vi "DropDetectionForLinkam.vi"(6 "Max(µm)":dbl min=0.0 format="%#_g µm", 7 "Min(µm)":dbl min=0.0 format="%#_g µm", 8 "error in":errorcluster, 9 "Mag":T1, 10 "Minimum match score":dbl=950.0, 11 "Image in":T4(plugin-control)) -> (0 "error out":errorcluster, 1 "Mag out":T1, 2 "Matches (pixel)":T3(array[cluster]), 3 "Image Out":T4(plugin-control), 4 "Circles (Calibrated)":T5(array[cluster]) {"Position"."Y" format="%.2f"; "Position"."X" format="%.2f"})   [LabVIEW 2013]
uses:
  Mag.ctl
  <vilib>/vision/NI_Vision_Development_Module.lvlib
  <vilib>/Analysis/NI_AALPro.lvlib
  <vilib>/Analysis/NI_AAL_SigProc.lvlib
panel:
  in  "Magnification (Microns/Pixel)":dbl(ring)=2.731524 items=["5x_M_BD"=2.731524, "10x_M"=1.3634, "10xM_BD"=1.3543, "10x_ph1"=1.3439, "20x_S"=0.68129, "20x_LM"=0.714285, "50x_S"=0.277777, "100x_im"=0.119047]
  out "fractional index or x":dbl
  out "XY Graph":cluster{i32[], "dX/dt":dbl[]}[](graph)
  in  "Annulus":T2 {"End Angle" min=-90.0 max=90.0 step=1.0 format="%.2f"; "Start Angle" min=-90.0 max=90.0 step=1.0 format="%.2f"; "Center X" scale=0.0..1024.0}
  in  "Circle Descriptor":cluster{"Min Radius":dbl, "Max Radius":dbl}={"Min Radius"=3.0, "Max Radius"=500.0}
  out "Number of matches":i32
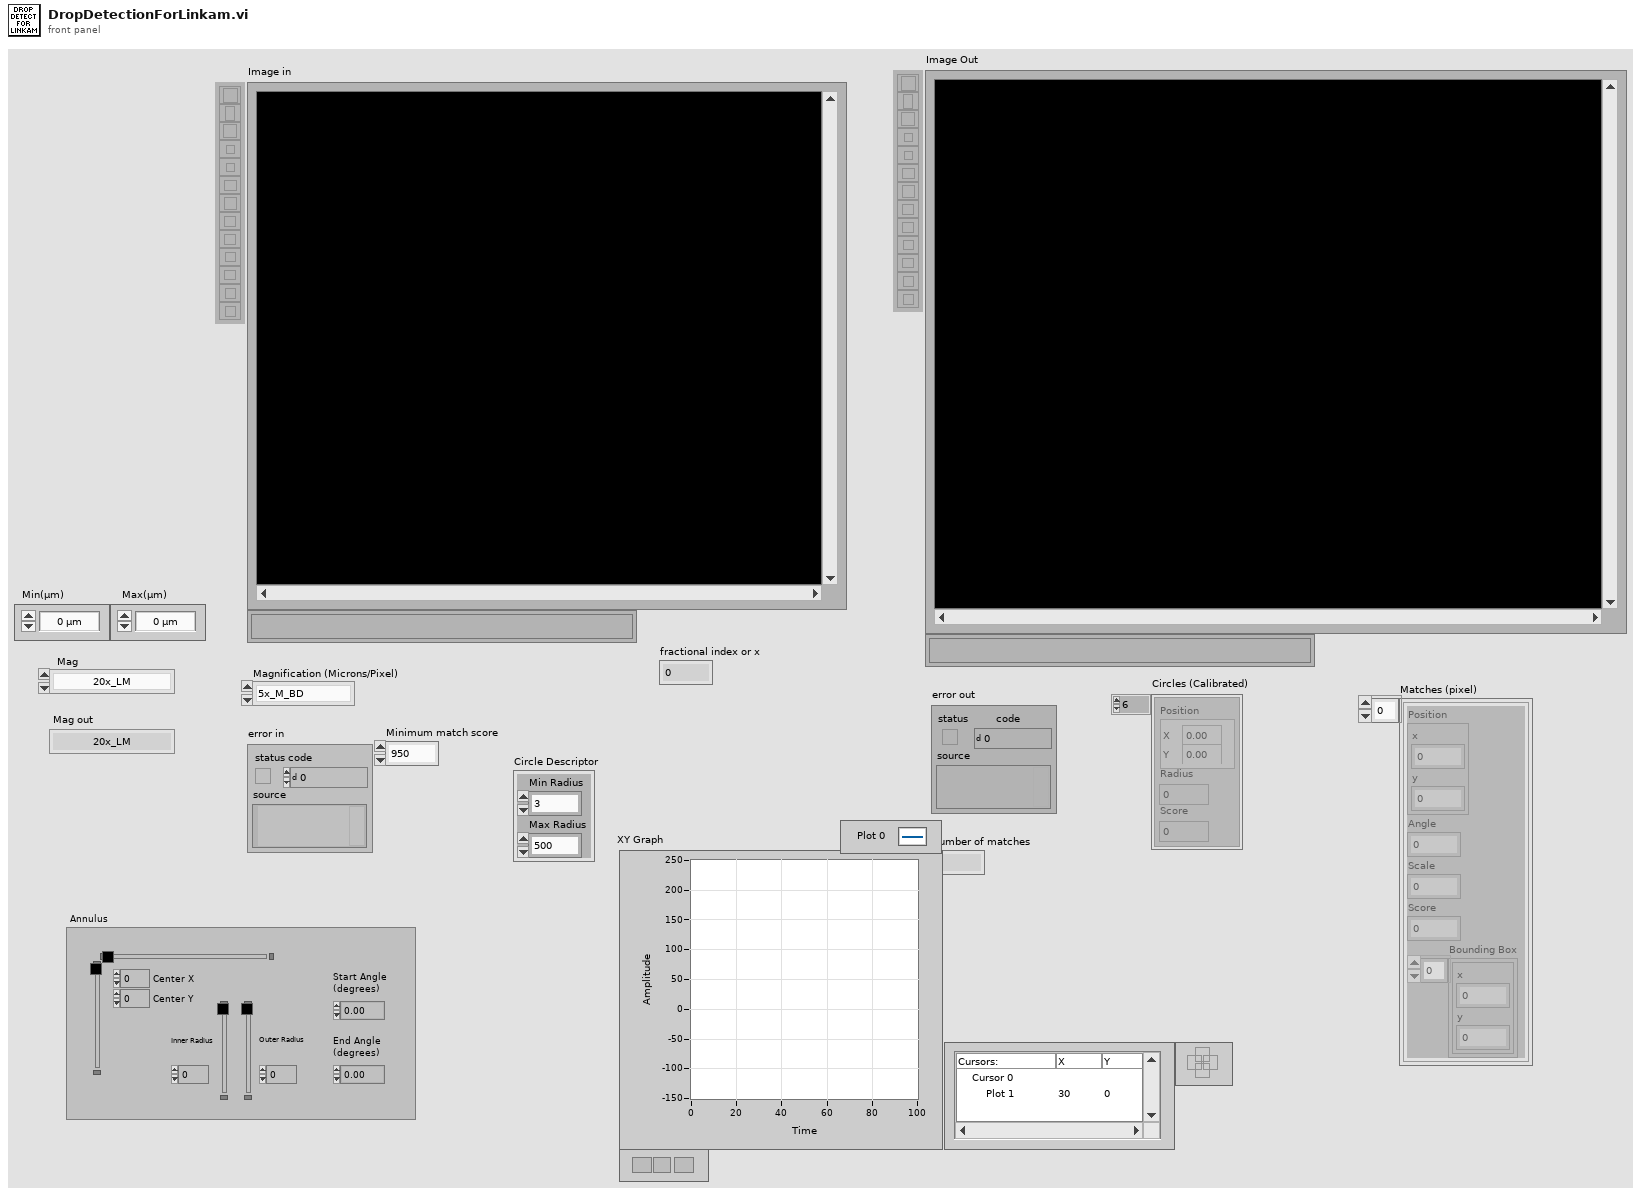
[diagram p1: front panel]
types:
  T1 = typedef "Mag.ctl" = enum16{"20x_LM", "50x_S", "100x_im"}
  T2 = typedef "IMAQ Circle" = cluster{"Center X":i32, "Center Y":i32, "Inner Radius":i32, "Outer Radius":i32, "Start Angle":dbl, "End Angle":dbl}
  T3 = cluster{"Position":cluster{"x":sgl, "y":sgl}, "Angle":sgl, "Scale":sgl, "Score":sgl, "Bounding Box":cluster{"x":sgl, "y":sgl}[]}[]
  T4 = typedef "IMAQ Image.ctl" = refnum<image>
  T5 = cluster{"Position":cluster{"X":sgl, "Y":sgl}, "Radius":dbl, "Score":dbl}[]
  T6 = cluster{"Extraction Mode":u32, "Edge Threshold":i32, "Edge Filter Size":u32, "Min Length":i32, "Row Search Step Size":i32, "Col Search Step Size":i32, "Max Endpoint Gap":i32, "Closed":bool, "Subpixel":bool}
  T7 = cluster{"Rotation":bool, "Scale":bool, "Occlusion":bool, "Range Settings":cluster{"Match Constraints":u32, "Min":dbl, "Max":dbl}[]}
  T8 = cluster{"Global Rectangle":i32[], "Contours":cluster{"ID":enum32{"External", "Internal"}, "Type":u32, "Coordinates":i32[]}[]}
  T9 = typedef "ROI Descriptor" = cluster{"Global Rectangle":i32[], "Contours":cluster{"ID":enum32{"External", "Internal"}, "Type":u32, "Coordinates":i32[]}[]}
  T10 = cluster{"Min":sgl, "Max":sgl, "Mean":sgl, "Std Dev":sgl, "Count":i32}
  T11 = cluster{"Position":cluster{"X":sgl, "Y":sgl}, "Radius":dbl, "Score":dbl}
  T12 = cluster{"Position":cluster{"x":sgl, "y":sgl}, "Angle":sgl, "Scale":sgl, "Score":sgl, "Bounding Box":cluster{"x":sgl, "y":sgl}[]}
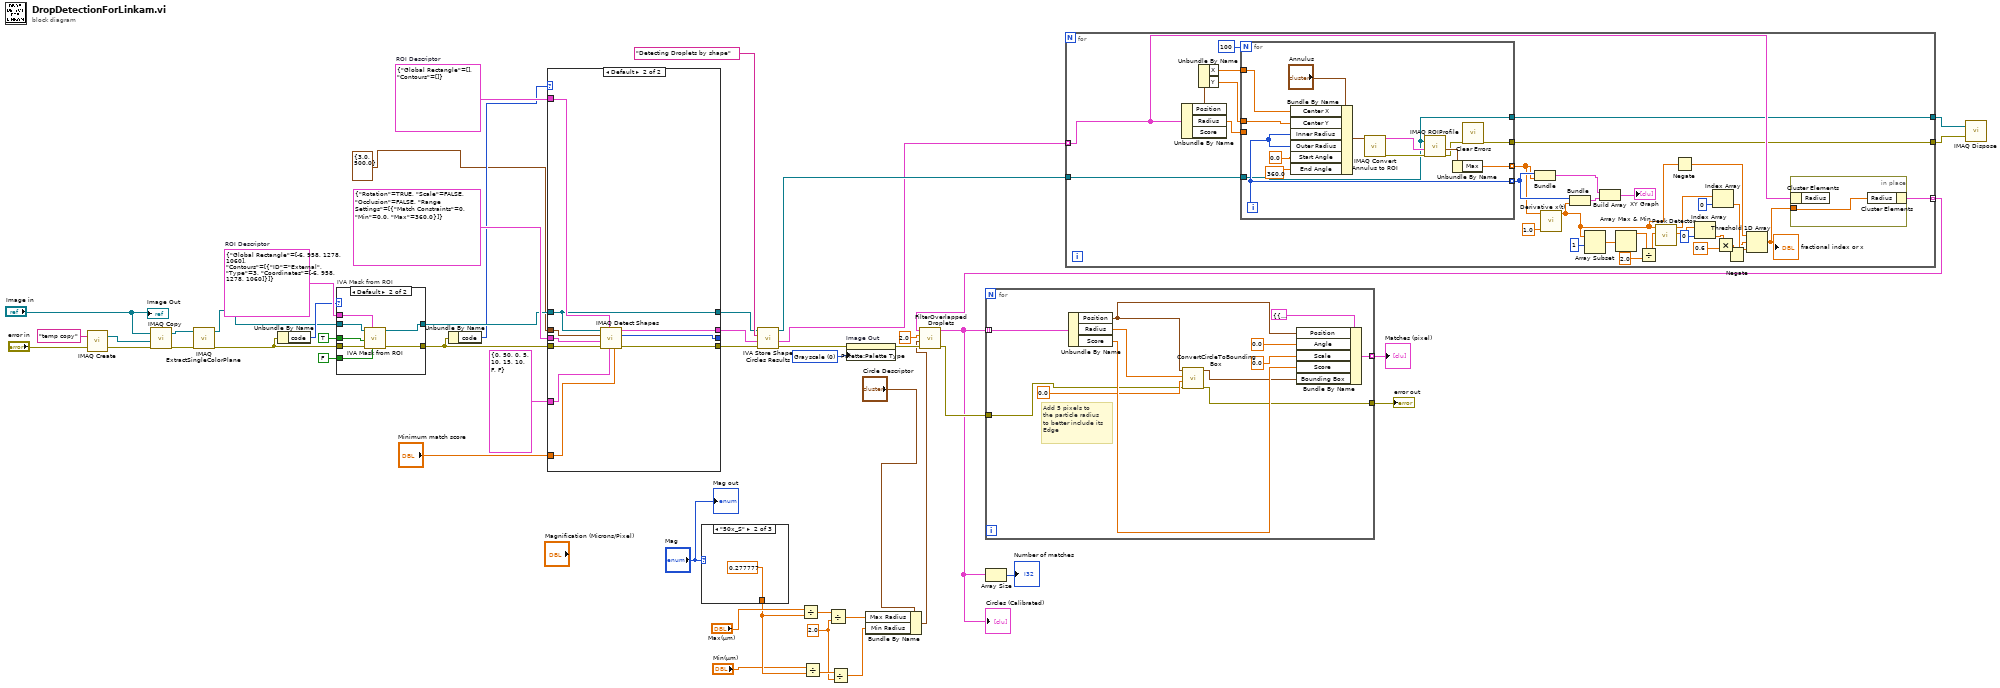
[diagram p0: block diagram]
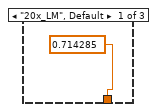
[diagram p2: hidden frame]
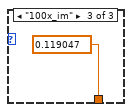
[diagram p3: hidden frame]
diagram:
  w17 = 2.0 ("y")
  w36 = u32 0 items=["Grayscale", "Binary", "Gradient", "Rainbow", "Temperature", "User Defined"] ("Palette")
  w44 = T8 {"Global Rectangle"=[], "Contours"=[]}  # ROI Descriptor
  w50 = T8 {"Global Rectangle"=[-6, 958, 1278, 1060], "Contours"=[{"ID"=enum."External", "Type"=3, "Coordinates"=[-6, 958, 1278, 1060]}]}  # ROI Descriptor
  n1 = call "IMAQ Create"("Image Name"="temp copy", "error in (no error)"="error in") -> ("New Image"=w12:T4, "error out"=w10:errorcluster)  [unwired: 2 in, 1 out]
  n2 = call "IMAQ Copy"("error in (no error)"=w10, "Image Dst"=w12, "Image Src"="Image in") -> ("error out"=w2:errorcluster, "Image Dst Out"=w4:T4)  [unwired: 3 in]
  n3 = call "IMAQ ExtractSingleColorPlane"("error in (no error)"=w2, "Image Src"=w4) -> ("error out"=w1:errorcluster, "Image Dst Out"=w3:T4)  [unwired: 8 in]
  n4 = Unbundle By Name(w1) -> ("code"=w47:i32)
  n5 = case "IVA Mask from ROI" shown="Default" w47 {
    tunnel: w50 -> [_ w58]
    tunnel: FALSE ("Shrink") -> [_ w57]
    tunnel: w3 -> [w51 w56]
    tunnel: w1 -> [_ w55]
    tunnel: [_ w54] -> w39
    tunnel: [w51 w53] -> w42
    tunnel: TRUE ("Out / In") -> [_ w52]
    frame -1074396199, -1074396198 {
      # "Discard\nCoordinate\nSystem\nError"
    }
    frame Default {
      n6 = call <vilib>:"IVA Mask from ROI.vi"("Shrink"=w57, "ROI Descriptor"=w58, "error in (no error)"=w55, "Out / In"=w52, "Image Src"=w56) -> ("error out"=w54:errorcluster, "Image Out"=w53:T4)  [unwired: 5 out]
    }
  }
  n7 = Unbundle By Name(w39) -> ("code"=w38:i32)
  n8 = case shown="Default" w38 {
    tunnel: w39 -> [_ w69]
    tunnel: [_ w68] -> _
    tunnel: T7 {"Rotation"=TRUE, "Scale"=FALSE, "Occlusion"=FALSE, "Range Settings"=[{"Match Constraints"=0, "Min"=0.0, "Max"=360.0}]} ("Match Options") -> [_ w67]
    tunnel: T6 {"Extraction Mode"=0, "Edge Threshold"=50, "Edge Filter Size"=0, "Min Length"=5, "Row Search Step Size"=10, "Col Search Step Size"=15, "Max Endpoint Gap"=10, "Closed"=FALSE, "Subpixel"=FALSE} ("Curve Parameters") -> [_ w66]
    tunnel: "Minimum match score" -> [_ w65]
    tunnel: cluster{"Min Radius":dbl, "Max Radius":dbl} {"Min Radius"=3.0, "Max Radius"=500.0} ("Circle Descriptor") -> [_ w64]
    tunnel: w44 -> [_ w63]
    tunnel: [_ w62] -> w43
    tunnel: w42 -> [w59 w60]
    tunnel: [_ w61] -> w41
    tunnel: [w59 w60] -> w37
    frame -1074396199, -1074396198 {
      # "Discard Coordinate\nSystem Error"
    }
    frame Default {
      n9 = call-poly "IMAQ Detect Shapes"("Minimum match score"=w65, "Curve Parameters"=w66, "ROI Descriptor"=w63, "error in (no error)"=w69, "Match Options"=w67, "Circle Descriptor"=w64, "Image"=w60) -> ("error out"=w61:errorcluster, "Number of Matches Returned"=w68:i32, "Circles"=w62:T5)  [unwired: 2 out]
    }
  }
  n10 = case shown="\"50x_S\"" "Mag" {
    tunnel: [w70 w71 w72] -> w21
    frame "20x_LM", Default {
      w70 = 0.714285 items=["5x_M_BD"=2.731524, "10x_M"=1.3634, "10xM_BD"=1.3543, "10x_ph1"=1.3439, "20x_S"=0.68129, "20x_LM"=0.714285, "50x_S"=0.277777, "100x_im"=0.119047] ("Magnification (Microns/Pixel)")
    }
    frame "50x_S" {
      w71 = 0.277777 items=["5x_M_BD"=2.731524, "10x_M"=1.3634, "10xM_BD"=1.3543, "10x_ph1"=1.3439, "20x_S"=0.68129, "20x_LM"=0.714285, "50x_S"=0.277777, "100x_im"=0.119047] ("Magnification (Microns/Pixel)")
    }
    frame "100x_im" {
      w72 = 0.119047 items=["5x_M_BD"=2.731524, "10x_M"=1.3634, "10xM_BD"=1.3543, "10x_ph1"=1.3439, "20x_S"=0.68129, "20x_LM"=0.714285, "50x_S"=0.277777, "100x_im"=0.119047] ("Magnification (Microns/Pixel)")
    }
  }
  n11 = call <vilib>:"IVA Store Shape Circles Results.vi"("error in (no error)"=w41, "Circles"=w43, "Step Name"="Detecting Droplets by shape", "Image in"=w37) -> ("error out"=w35:errorcluster, "Circles (Calibrated)"=w25:T5, "Image dup"=w26:T4)  [unwired: 5 out]
  n12 = Divide(x="Max(µm)", y=w21) -> (x/y=w19:dbl)
  n13 = Divide(x="Min(µm)", y=w21) -> (x/y=w18:dbl)
  n14 = Divide(x=w19, y=w17) -> (x/y=w15:dbl)
  n15 = Divide(x=w18, y=w17) -> (x/y=w14:dbl)
  n16 = property on="Image Out" class="ImageControl"(error in=w35, "Palette:Palette Type"=w36) -> (error out=w30:errorcluster)  [unwired: 1 in, 1 out]
  n17 = Bundle By Name(cluster="Circle Descriptor", "Max Radius"=w15, "Min Radius"=w14) -> (w13:cluster{"Min Radius":dbl, "Max Radius":dbl})
  n18 = for {
    tunnel: w26 -> [w105]
    tunnel: w25 -> [w86] mode=indexing
    tunnel: [w85] -> w24 mode=indexing
    tunnel: [w74] -> w6
    tunnel: [w73] -> w7
    n19 = Unbundle By Name(w86) -> ("Position"=w104:cluster{"X":sgl, "Y":sgl}, "Radius"=w87:dbl)  [unwired: 1 out]
    n20 = Unbundle By Name(w104) -> ("X"=w103:sgl, "Y"=w102:sgl)
    n21 = for {
      N: 100 -> [_]
      tunnel: w105 -> [w107]
      tunnel: w87 -> [_]
      tunnel: w103 -> [w117]
      tunnel: w102 -> [w116]
      tunnel: [w112] -> w99 mode=indexing
      tunnel: [w110] -> w100 mode=indexing
      tunnel: [w108] -> w74
      tunnel: [w107] -> w73
      i -> [w110]
      n22 = Bundle By Name(cluster="Annulus", "Center X"=w117, "Center Y"=w116, "Inner Radius"=w110, "Outer Radius"=w110, "Start Angle"=0.0, "End Angle"=360.0) -> (w115:T2)
      n23 = call "IMAQ Convert Annulus to ROI"("Annulus"=w115) -> ("error out"=w114:errorcluster, "ROI Descriptor"=w120:T9)  [unwired: 8 in]
      n24 = call "IMAQ ROIProfile"("error in (no error)"=w114, "ROI Descriptor"=w120, "Image"=w107) -> ("ROI Pixel Statistics"=w113:T10, "error out"=w109:errorcluster)  [unwired: 1 in, 3 out]
      n25 = Unbundle By Name(w113) -> ("Max"=w112:sgl)
      n26 = call <vilib>:"Clear Errors.vi"("error in (no error)"=w109) -> ("error out"=w108:errorcluster)  [unwired: 6 in]
    }
    n27 = Bundle(w100, w99) -> (w98:cluster{i32[], sgl[]})  [unwired: 1 in]
    n28 = call <vilib>:"Derivative x(t).vi"("dt"=1.0, "X"=w99) -> ("dX/dt"=w79:dbl[])  [unwired: 8 in, 1 out]
    n29 = Bundle(w100, "dX/dt"=w79) -> (w97:cluster{i32[], "dX/dt":dbl[]})  [unwired: 1 in]
    n30 = Array Subset(array=w79, index=1) -> (w93:dbl[])  [unwired: 1 in]
    n31 = Build Array(w98, w97) -> (→"XY Graph":cluster{i32[], "dX/dt":dbl[]}[])
    n32 = Array Max & Min(array=w93) -> (max value=w92:dbl)  [unwired: 3 out]
    n33 = Divide(x=w92, y=2.0) -> (x/y=w90:dbl)
    n34 = call <vilib>:"Peak Detector.vi"("threshold"=w90, "X"=w79) -> ("Amplitudes"=w82:dbl[], "Locations"=w89:dbl[])  [unwired: 5 in, 3 out]
    n35 = Negate(x=w79) -> (-x=w78:dbl[])
    n36 = Index Array(array=w82, index=0) -> (element=w80:dbl)
    n37 = Index Array(array=w89, index=0) -> (element=w84:dbl)
    n38 = Multiply(x=w80, y=0.6) -> (x*y=w77:dbl)
    n39 = Negate(x=w77) -> (-x=w76:dbl)
    n40 = Threshold 1D Array(1:w84, 2:w76, 3:w78) -> (0:w75:dbl)
    "fractional index or x" <- w75
    n41 = in-place {
      in-place-border: w75 -> [w106]
      n42 = in-place-cluster #1(w86) -> ()  [unwired: 1 out]
      n43 = in-place-cluster #1("Radius"=w106) -> (w85:T11)
    }
  }
  n44 = call "FilterOverlappedDroplets.vi"("error in (no error)"=w30, "Circle Descriptor"=w13, "Threshold (pixels)"=2.0, "Circles (Calibrated)"=w24) -> ("error out"=w28:errorcluster, "Circles (Calibrated) 2"=w23:T5)  [unwired: 6 in]
  "Circles (Calibrated)" <- w23
  n45 = for {
    tunnel: w23 -> [w131] mode=indexing
    tunnel: [w127] -> w32 mode=indexing
    tunnel: w28 -> [w122]
    tunnel: [w121] -> w27
    # "Add 5 pixels to\nthe particle radius \nto better include its\nEdge"
    n46 = Unbundle By Name(w131) -> ("Position"=w125:cluster{"X":sgl, "Y":sgl}, "Radius"=w124:dbl, "Score"=w130:dbl)
    n47 = call "ConvertCircleToBoundingBox.vi"("error in (no error)"=w122, "InflateBoxbyPixelNo"=0.0 ("y"), "Radius"=w124, "Position"=w125) -> ("error out"=w121:errorcluster, "Bounding Box"=w126:cluster{"x":sgl, "y":sgl}[])  [unwired: 6 in]
    n48 = Bundle By Name(cluster=T12 {"Position"={"x"=0.0, "y"=0.0}, "Angle"=0.0, "Scale"=0.0, "Score"=0.0, "Bounding Box"=[]} ("element"), "Position"=w125, "Angle"=sgl 0.0, "Scale"=sgl 0.0, "Score"=w130, "Bounding Box"=w126) -> (w127:T12)
  }
  "error out" <- w27
  "Matches (pixel)" <- w32
  n49 = Array Size(array=w23) -> (size(s)=→"Number of matches":i32)
  n50 = call "IMAQ Dispose"("Image"=w7, "error in (no error)"=w6) -> ()  [unwired: 4 in, 1 out]
  "Image Out" <- "Image in"
  "Mag out" <- "Mag"
